vi "wfsizecalc.vi"(0 "Sampling frequency (Hz)":dbl, 1 "AOtab":i32, 2 "reference waveforms to":string, 3 "channel":string, 5 "Repeats":dbl, 9 "Cycles":dbl, 10 "Matlab wave file":path, 11 "pulses":dbl, 12 "Period (ms)":dbl, 14 "Frequency":dbl, 15 "Tri Repeats":dbl) -> (4 "total size GB":dbl, 6 "gigabytesize wf":dbl)   [LabVIEW 2015]
uses:
  <vilib>/Utility/file.llb/Read Delimited Spreadsheet (DBL).vi
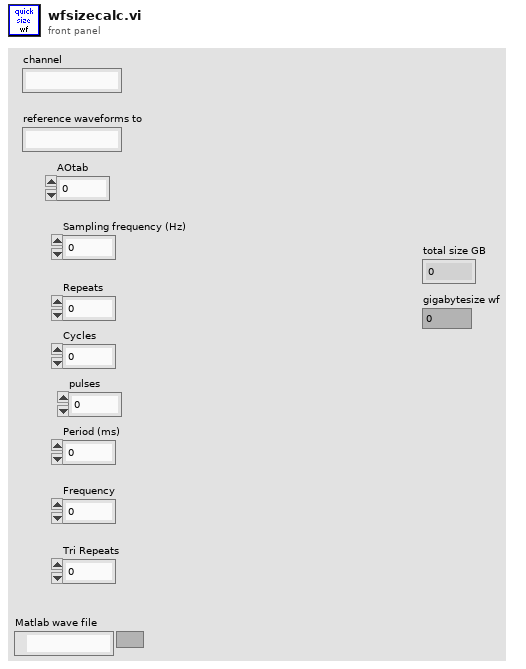
[diagram p1: front panel]
types:
  T1 = cluster{"AO parameters":cluster{"AOtab":dbl, "Repeats":dbl, "Cycles":dbl, "Start amplitude (V)":dbl, "Baseline (V)":dbl, "Step size (V)":dbl, "DC (%)":dbl, "Sampling frequency (Hz)":dbl, "Period (ms)":dbl, "Offset (V)":dbl, "Amplitude (V)":dbl, "Frequency":dbl, "Tri Repeats":dbl, "phase shift (ms)":dbl, "Pulses":dbl, "Matlab wave file":path, "Tri phase":dbl, "padding value":dbl}[], "DO parameters":cluster{"Digital DC (%)":dbl, "Digital phase":dbl, "Digital Freq (Hz)":dbl, "Sampling frequency (Hz)":dbl, "Digital time offset (s) ":dbl, "padding value":dbl, "matlab wave file":path, "DOtab":dbl}[]}
  T2 = cluster{"AOtab":dbl, "Repeats":dbl, "Cycles":dbl, "Start amplitude (V)":dbl, "Baseline (V)":dbl, "Step size (V)":dbl, "DC (%)":dbl, "Sampling frequency (Hz)":dbl, "Period (ms)":dbl, "Offset (V)":dbl, "Amplitude (V)":dbl, "Frequency":dbl, "Tri Repeats":dbl, "phase shift (ms)":dbl, "Pulses":dbl, "Matlab wave file":path, "Tri phase":dbl, "padding value":dbl}[]
  T3 = cluster{"AOtab":dbl, "Repeats":dbl, "Cycles":dbl, "Start amplitude (V)":dbl, "Baseline (V)":dbl, "Step size (V)":dbl, "DC (%)":dbl, "Sampling frequency (Hz)":dbl, "Period (ms)":dbl, "Offset (V)":dbl, "Amplitude (V)":dbl, "Frequency":dbl, "Tri Repeats":dbl, "phase shift (ms)":dbl, "Pulses":dbl, "Matlab wave file":path, "Tri phase":dbl, "padding value":dbl}
  T4 = cluster{"Digital DC (%)":dbl, "Digital phase":dbl, "Digital Freq (Hz)":dbl, "Sampling frequency (Hz)":dbl, "Digital time offset (s) ":dbl, "padding value":dbl, "matlab wave file":path, "DOtab":dbl}[]
  T5 = cluster{"Digital DC (%)":dbl, "Digital phase":dbl, "Digital Freq (Hz)":dbl, "Sampling frequency (Hz)":dbl, "Digital time offset (s) ":dbl, "padding value":dbl, "matlab wave file":path, "DOtab":dbl}
  T6 = typedef "LVRectTypeDef.ctl" = cluster{"Left":i16, "Top":i16, "Right":i16, "Bottom":i16}
  T7 = cluster{"Xpixels":i32, "Vxminref":dbl, "Vxmaxref":dbl, "P":dbl, "Ypixels":i32, "Vyminref":dbl, "Vymaxref":dbl, "srate":sgl, "sAOxy":i32, "timeout":dbl, "type":string, "date":string, "time":string, "Colormap":u16, "Drawing Mode":u16, "Scanning Mode":u16, "square pixels":bool, "square matrix":bool, "Xpixels Img":i32, "Vx-min Img":dbl, "VX-max Img":dbl, "Ypixels Img":i32, "Vy-min Img":dbl, "Vy-max Img ":dbl, "Angle Img":dbl, "autoshutter":bool, "finite":bool, "cont":bool, "wavdet":bool, "measpoints":i32, "avpp":i32, "bufferAO":i32, "bufferAI":i32, "starttick":u32, "waveform":path, "Vx-ref":dbl, "Vy-ref":dbl, "refreshrate":dbl, "refreshbuffer":i32, "tt_cycles":i32, "motorref":refnum<k7>, "mirrorswitch":refnum<k7>, "sample mode":i32, "maxbufferAI":i32, "srateAODO":sgl, "bin":sgl, "Pel":sgl, "Angle draw":dbl, "srate Img":sgl, "ROIimg_plotbounds":T6, "auto OD":bool, "ODfilt":u16, "aAI":i32[], "aCI":i32[], "aAO":u32[], "aDO":u32[], "refwfsize":dbl, "Lifetime":bool, "Vz-Img":dbl, "Vz-ref":dbl, "Vz-reset":dbl, "AIoverride":bool, "aAS":u32[], "XYZstart":dbl[]}
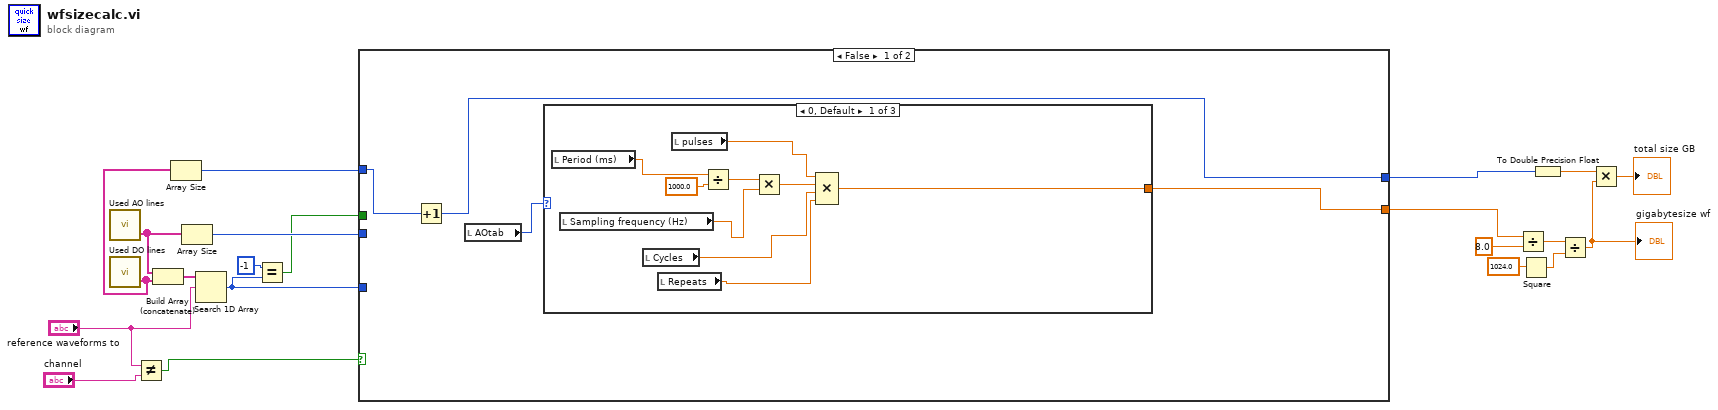
[diagram p0: block diagram]
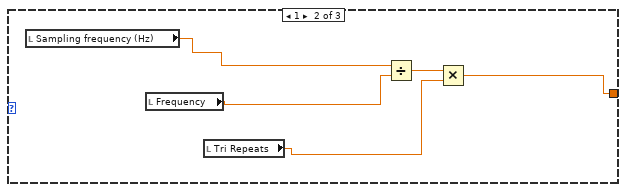
[diagram p2: hidden frame]
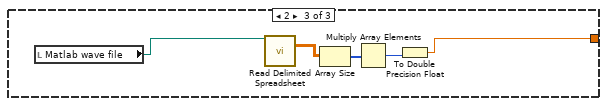
[diagram p3: hidden frame]
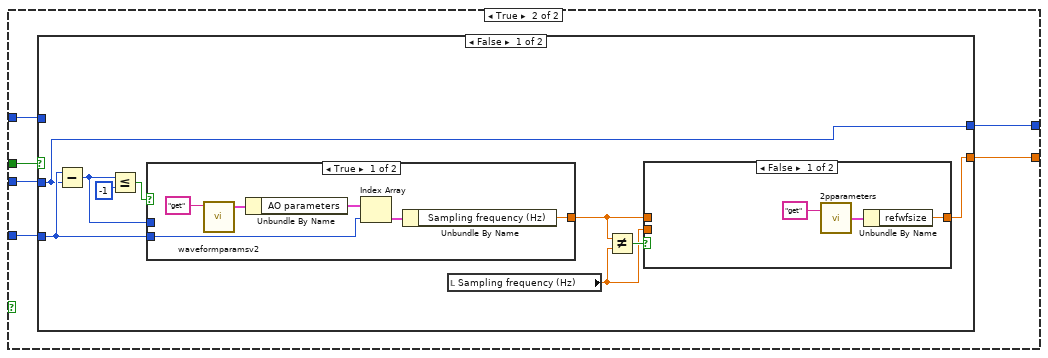
[diagram p4: hidden frame]
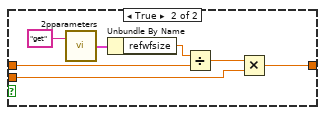
[diagram p5: hidden frame]
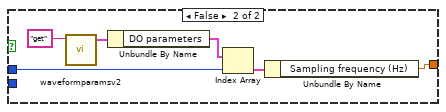
[diagram p6: hidden frame]
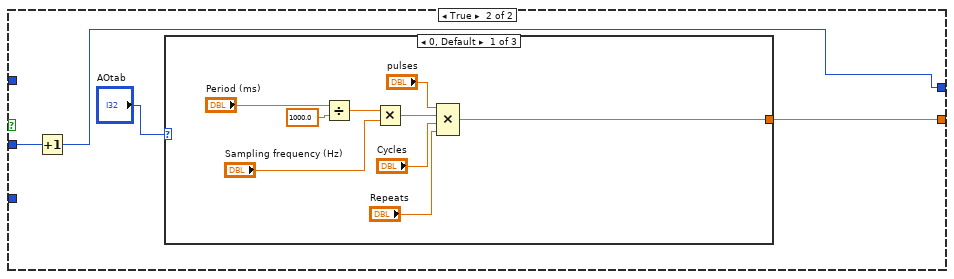
[diagram p7: hidden frame]
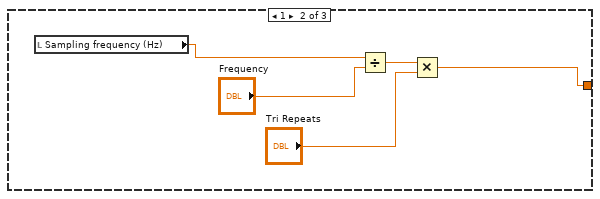
[diagram p8: hidden frame]
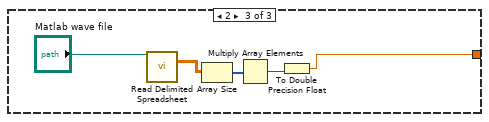
[diagram p9: hidden frame]
diagram:
  n1 = call "Used AO lines.vi"() -> ("used AO names"=w19:string[])  [unwired: 2 in, 1 out]
  n2 = call "Used DO lines.vi"() -> ("used DO names"=w9:string[])  [unwired: 2 in, 1 out]
  n3 = Not Equal?(x="reference waveforms to", y="channel") -> (x != y?=w1:bool)
  n4 = Build Array (concatenate)(w19, w9) -> (w18:string[])
  n5 = Array Size(array=w9) -> (size(s)=w8:i32)
  n6 = Array Size(array=w19) -> (size(s)=w20:i32)
  n7 = Search 1D Array(1D array=w18, element="reference waveforms to") -> (index of element=w17:i32)  [unwired: 1 in]
  n8 = Equal?(x=-1, y=w17) -> (x = y?=w15:bool)
  n9 = case shown="False" w1 {
    tunnel: w20 -> [_ w49]
    tunnel: w17 -> [_ w48]
    tunnel: w15 -> [_ w47]
    tunnel: [w22 w46] -> w12
    tunnel: w8 -> [w24 w45]
    tunnel: [w23 w44] -> w7
    frame False {
      n10 = Increment(x=w24) -> (x+1=w23:i32)
      n11 = local read "AOtab"() -> (w21:i32)
      n12 = case shown="0, Default" w21 {
        tunnel: [w30 w37 w40] -> w22
        frame 0, Default {
          n13 = local read "Period (ms)"() -> (w28:dbl)
          n14 = local read "Sampling frequency (Hz)"() -> (w27:dbl)
          n15 = local read "Cycles"() -> (w26:dbl)
          n16 = local read "Repeats"() -> (w25:dbl)
          n17 = local read "pulses"() -> (w29:dbl)
          n18 = Divide(x=w28, y=1000.0) -> (x/y=w32:dbl)
          n19 = Multiply(x=w32, y=w27) -> (x*y=w33:dbl)
          n20 = Compound Arithmetic op=MULTIPLY(w29, w33, w26, w25) -> (w30:dbl)
        }
        frame 1 {
          n21 = local read "Sampling frequency (Hz)"() -> (w36:dbl)
          n22 = local read "Frequency"() -> (w35:dbl)
          n23 = local read "Tri Repeats"() -> (w34:dbl)
          n24 = Divide(x=w36, y=w35) -> (x/y=w38:dbl)
          n25 = Multiply(x=w38, y=w34) -> (x*y=w37:dbl)
        }
        frame 2 {
          n26 = local read "Matlab wave file"() -> (w39:path)
          n27 = call-poly <vilib>:"Read Delimited Spreadsheet.vi"("file path (dialog if empty)"=w39) -> ("all rows"=w42:dbl[][])  [unwired: 9 in, 5 out]
          n28 = Array Size(array=w42) -> (size(s)=w41:i32[])
          n29 = Multiply Array Elements(1:w41) -> (0:w43:i32)
          n30 = To Double Precision Float(number=w43) -> (double precision float=w40:dbl)
        }
      }
    }
    frame True {
      n31 = case shown="False" w47 {
        tunnel: w49 -> [w50 w82]
        tunnel: w48 -> [w52 _]
        tunnel: [w51 w83] -> w46
        tunnel: w45 -> [_ _]
        tunnel: [w50 w81] -> w44
        frame False {
          n32 = Subtract(x=w52, y=w50) -> (x-y=w56:i32)
          n33 = Less Or Equal?(x=w56, y=-1) -> (x <= y?=w57:bool)
          n34 = case shown="True" w57 {
            tunnel: w52 -> [w71 _]
            tunnel: w56 -> [_ w76]
            tunnel: [w69 w75] -> w54
            frame True {
              n35 = call "waveformparamsv2.vi"("command"="get") -> ("Params out"=w74:T1)  [unwired: 4 in, 2 out]
              n36 = Unbundle By Name(w74) -> ("AO parameters"=w72:T2)
              n37 = Index Array(array=w72, index=w71) -> (element=w70:T3)
              n38 = Unbundle By Name(w70) -> ("Sampling frequency (Hz)"=w69:dbl)
            }
            frame False {
              n39 = call "waveformparamsv2.vi"("command"="get") -> ("Params out"=w80:T1)  [unwired: 4 in, 2 out]
              n40 = Unbundle By Name(w80) -> ("DO parameters"=w78:T4)
              n41 = Index Array(array=w78, index=w76) -> (element=w77:T5)
              n42 = Unbundle By Name(w77) -> ("Sampling frequency (Hz)"=w75:dbl)
            }
          }
          n43 = local read "Sampling frequency (Hz)"() -> (w53:dbl)
          n44 = Not Equal?(x=w54, y=w53) -> (x != y?=w55:bool)
          n45 = case shown="False" w55 {
            tunnel: w54 -> [_ w66]
            tunnel: w53 -> [_ w63]
            tunnel: [w59 w62] -> w51
            frame False {
              n46 = call "2pparameters.vi"("command"="get") -> ("params out"=w61:T7)  [unwired: 1 in]
              n47 = Unbundle By Name(w61) -> ("refwfsize"=w59:dbl)
            }
            frame True {
              n48 = call "2pparameters.vi"("command"="get") -> ("params out"=w68:T7)  [unwired: 1 in]
              n49 = Unbundle By Name(w68) -> ("refwfsize"=w65:dbl)
              n50 = Divide(x=w65, y=w66) -> (x/y=w64:dbl)
              n51 = Multiply(x=w64, y=w63) -> (x*y=w62:dbl)
            }
          }
        }
        frame True {
          n52 = Increment(x=w82) -> (x+1=w81:i32)
          n53 = case shown="0, Default" "AOtab" {
            tunnel: [w85 w94 w99] -> w83
            frame 0, Default {
              n54 = Divide(x="Period (ms)", y=1000.0) -> (x/y=w88:dbl)
              n55 = Multiply(x=w88, y="Sampling frequency (Hz)") -> (x*y=w91:dbl)
              n56 = Compound Arithmetic op=MULTIPLY("pulses", w91, "Cycles", "Repeats") -> (w85:dbl)
            }
            frame 1 {
              n57 = local read "Sampling frequency (Hz)"() -> (w98:dbl)
              n58 = Divide(x=w98, y="Frequency") -> (x/y=w96:dbl)
              n59 = Multiply(x=w96, y="Tri Repeats") -> (x*y=w94:dbl)
            }
            frame 2 {
              n60 = call-poly <vilib>:"Read Delimited Spreadsheet.vi"("file path (dialog if empty)"="Matlab wave file") -> ("all rows"=w101:dbl[][])  [unwired: 9 in, 5 out]
              n61 = Array Size(array=w101) -> (size(s)=w100:i32[])
              n62 = Multiply Array Elements(1:w100) -> (0:w103:i32)
              n63 = To Double Precision Float(number=w103) -> (double precision float=w99:dbl)
            }
          }
        }
      }
    }
  }
  n64 = Divide(x=w12, y=8.0) -> (x/y=w11:dbl)
  n65 = Square(x=1024.0 ("y")) -> (x^2=w10:dbl)
  n66 = To Double Precision Float(number=w7) -> (double precision float=w6:dbl)
  n67 = Divide(x=w11, y=w10) -> (x/y=w5:dbl)
  "gigabytesize wf" <- w5
  n68 = Multiply(x=w6, y=w5) -> (x*y=→"total size GB":dbl)
